vi "Read Key (Variant)__lvcfg.vi"(5 "format string (%;%f)":string="%f", 7 "section":string, 8 "error in (no error)":errorcluster, 9 "type":variant, 10 "key (optional)":string, 11 "Config in":T1) -> (0 "error out":errorcluster, 1 "key-value":variant, 2 "found?":bool, 3 "Config out":T1)   [LabVIEW 2017, in "LabVIEW Config(Variant).lvlib"]
doc: "Reads a value associated with key in a specified section of the configuration data identified by refnum. If \"key\" input is not specified, the name of the variant object is used as the key. the \"found?\" output will be TRUE for compount objects (clusters) only if all elements (recursively) are found.\n\nFor example a Boolean named \"Enable\" with a value of TRUE would correspond to the key-value pair:\n\nEnable=TRUE\n\nNote: Special characters in section and key names will be escape-coded. These include the following: \\00-\\1F (non-printable chars); \"[\", \"]\", and \"=\" (INI syntax elements); \\FE (\"þ\") and \\FF (\"ÿ\") (legacy bracket encoding); Additionally, the escape character, \"\\\", will be escaped as \"\\\\\"."
uses:
  LabVIEW Config(Variant).lvlib
  <userlib>/_NEVSTOP/Communicable State Machine(CSM)/addons/INI-Static-Variable-Support/LabVIEW-Config/Config.ctl
  <userlib>/_NEVSTOP/Communicable State Machine(CSM)/addons/INI-Static-Variable-Support/LabVIEW-Config/Read Key (String).vi
  <userlib>/_NEVSTOP/Communicable State Machine(CSM)/addons/INI-Static-Variable-Support/LabVIEW-Config/Read Key (Boolean).vi
  <userlib>/_NEVSTOP/Communicable State Machine(CSM)/addons/INI-Static-Variable-Support/LabVIEW-Config/Read Key (DBL).vi
  <userlib>/_NEVSTOP/Communicable State Machine(CSM)/addons/INI-Static-Variable-Support/LabVIEW-Config/Read Key (U32).vi
  <userlib>/_NEVSTOP/Communicable State Machine(CSM)/addons/INI-Static-Variable-Support/LabVIEW-Config/Read Key (I32).vi
  <userlib>/_NEVSTOP/Communicable State Machine(CSM)/addons/INI-Static-Variable-Support/LabVIEW-Config/LabVIEW-Config.lvlib
  <userlib>/_NEVSTOP/Communicable State Machine(CSM)/Communicable State Machine.lvlib
panel:
  in  "Ref for recursive call":refnum<vi>
  # "Read Key (Variant).vi\n\nReads a variant key-value from INI file.\n\nPlease visit http://www.OpenG.org to learn about the\nOpen Source LabVIEW software movement.\n\nNOTICE -- YOU MUST LEAVE THIS NOTICE IN PLACE.  PER THE TERMS OF THE LICENSE BELOW, YOU MAY SUBLICENSE THIS SOFTWARE \nIN ANY WAY THAT DOES NOT CONFLICT WITH THIS LICENSE.\n\n### BSD License (http://www.opensource.org/licenses/bsd-license.php) Begin ###\n \nCopyright (c) 2002, Jean-Pierre Drolet <drolet_jp@hotmail.com>\nCopyright (c) 2002-2006, Jim Kring <jim@jimkring.com>\n\nAll rights reserved.\n\nRedistribution and use in source and binary forms, with or without modification, are permitted provided that the following conditions are met:\n\n    * Redistributions of source code must retain the above copyright notice, this list of conditions and the following disclaimer.\n    * Redistributions in binary form must reproduce the above copyright notice, this list of conditions and the following disclaimer in the \n       documentation and/or other materials provided with the distribution.\n    * Neither the name of SciWare, James Kring, Inc., nor the names of its contributors may be used to endorse or promote products derived \n       from this software without specific prior written permission.\n\nTHIS SOFTWARE IS PROVIDED BY THE COPYRIGHT HOLDERS AND CONTRIBUTORS \"AS IS\" AND ANY EXPRESS OR IMPLIED WARRANTIES, \nINCLUDING, BUT NOT LIMITED TO, THE IMPLIED WARRANTIES OF MERCHANTABILITY AND FITNESS FOR A PARTICULAR PURPOSE ARE \nDISCLAIMED. IN NO EVENT SHALL THE COPYRIGHT OWNER OR CONTRIBUTORS BE LIABLE FOR ANY DIRECT, INDIRECT, INCIDENTAL,\n SPECIAL, EXEMPLARY, OR CONSEQUENTIAL DAMAGES (INCLUDING, BUT NOT LIMITED TO, PROCUREMENT OF SUBSTITUTE GOODS OR \nSERVICES; LOSS OF USE, DATA, OR PROFITS; OR BUSINESS INTERRUPTION) HOWEVER CAUSED AND ON ANY THEORY OF LIABILITY, \nWHETHER IN CONTRACT, STRICT LIABILITY, OR TORT (INCLUDING NEGLIGENCE OR OTHERWISE) ARISING IN ANY WAY OUT OF THE USE \nOF THIS SOFTWARE, EVEN IF ADVISED OF THE POSSIBILITY OF SUCH DAMAGE.\n\n### BSD License End ###"
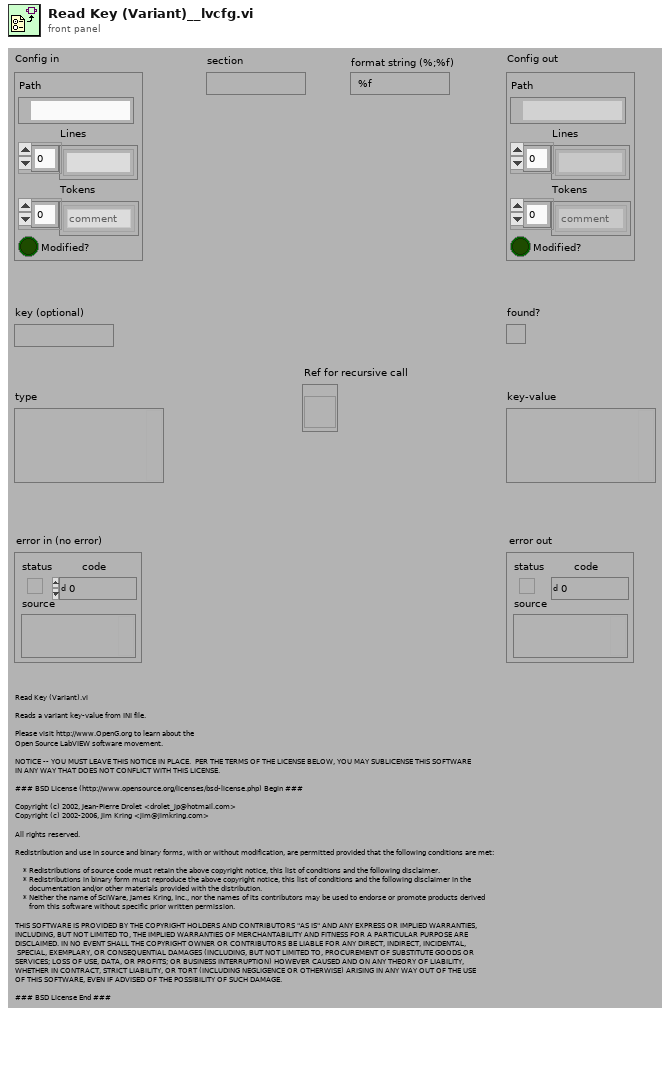
[diagram p1: front panel]
types:
  T1 = typedef "LabVIEW-Config.lvlib/Config.ctl" = cluster{"Path":path, "Lines":string[], "Tokens":enum8{"comment", "section", "key"}[], "Modified?":bool}
  T2 = typedef "Type Descriptor Enumeration__ogtk.ctl" = enum8{"<Null>", "I8", "I16", "I32", "I64", "U8", "U16", "U32", "U64", "SGL", "DBL", "EXT", "CSG", "CDB", "CXT", "0x0F", "0x10", "0x11", "0x12", "0x13", "0x14", "Enum U8", "Enum U16", "Enum U32", "Enum U64", "SGL PQ", "DBL PQ", "EXT PQ", "CSG PQ", "CDB PQ", "CXT PQ", "0x1F", "0x20", "Boolean", "0x22", "0x23", "0x24", "0x25", "0x26", "0x27", "0x28", "0x29", "0x2A", "0x2B", "0x2C", "0x2D", "0x2E", "0x2F", "String", "0x31", "Path", "Pict", "0x34", "0x35", "0x36", "DAQ", "0x38", "0x39", "0x3A", "0x3B", "0x3C", "0x3D", "0x3E", "0x3F", "Array", "0x41", "0x42", "0x43", "0x44", "0x45", "0x46", "0x47", "0x48", "0x49", "0x4A", "0x4B", "0x4C", "0x4D", "0x4E", "0x4F", "Cluster", "0x51", "0x52", "Variant", "Waveform", "0x55", "0x56", "0x57", "0x58", "0x59", "0x5A", "0x5B", "0x5C", "0x5D", "0x5E", "Fixed Point", "0x60", "0x61", "0x62", "0x63", "0x64", "0x65", "0x66", "0x67", "0x68", "0x69", "0x6A", "0x6B", "0x6C", "0x6D", "0x6E", "0x6F", "Refnum", "0x71", "0x72", "Set Collection", "Map Collection"}
  T3 = typedef "Type Descriptor__ogtk.ctl" = i16[]
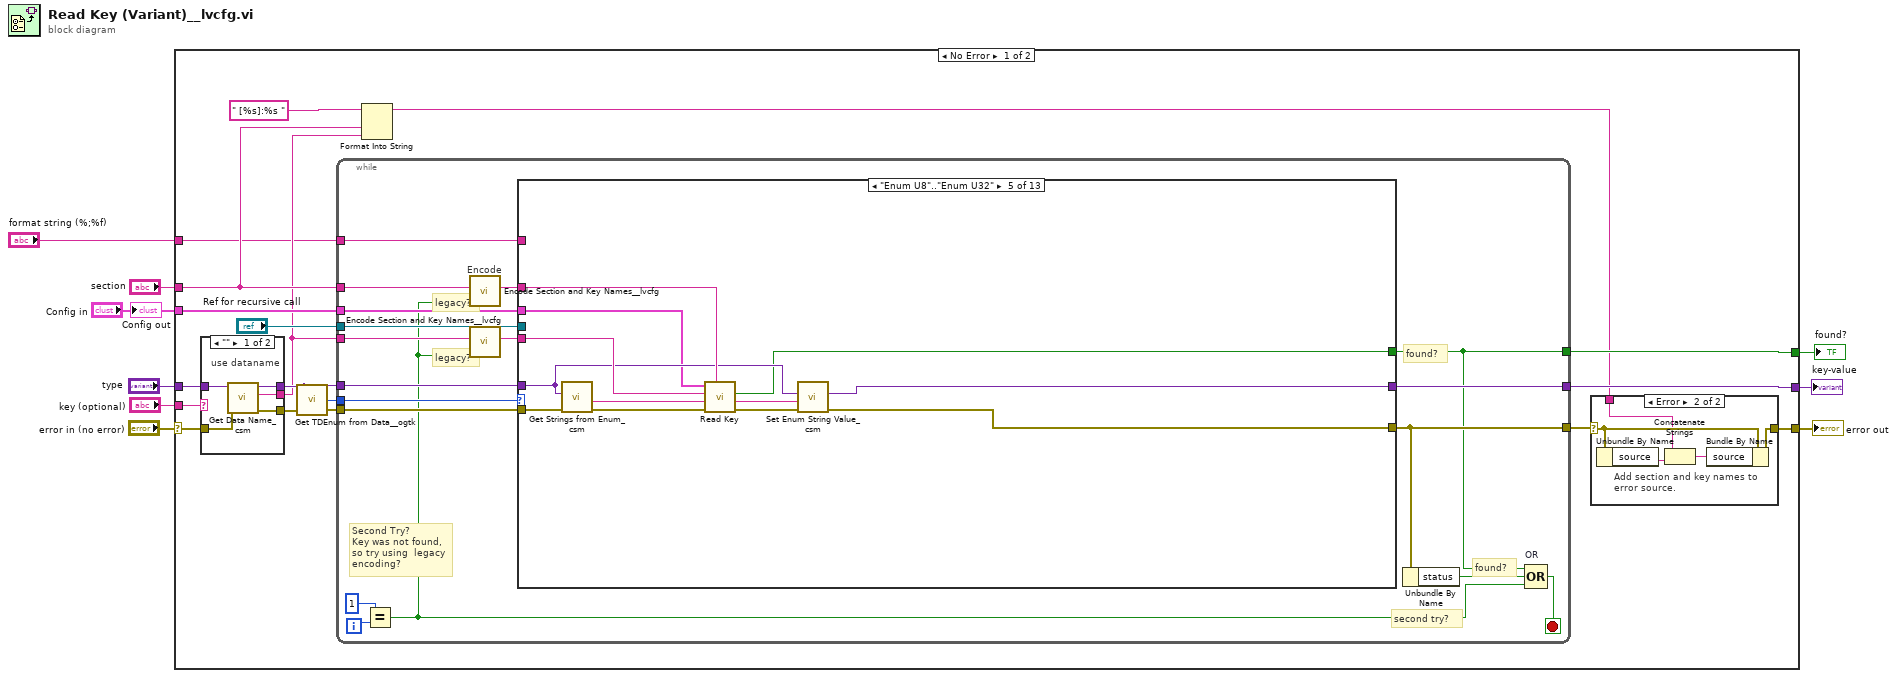
[diagram p0: block diagram]
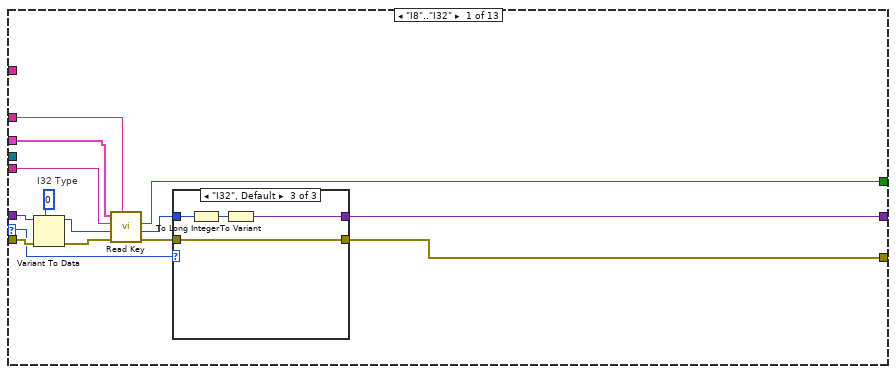
[diagram p2: hidden frame]
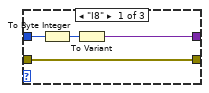
[diagram p3: hidden frame]
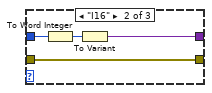
[diagram p4: hidden frame]
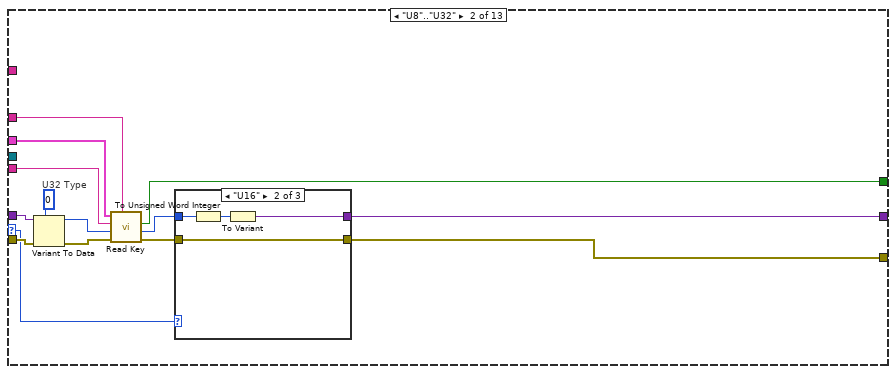
[diagram p5: hidden frame]
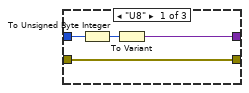
[diagram p6: hidden frame]
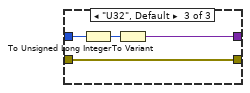
[diagram p7: hidden frame]
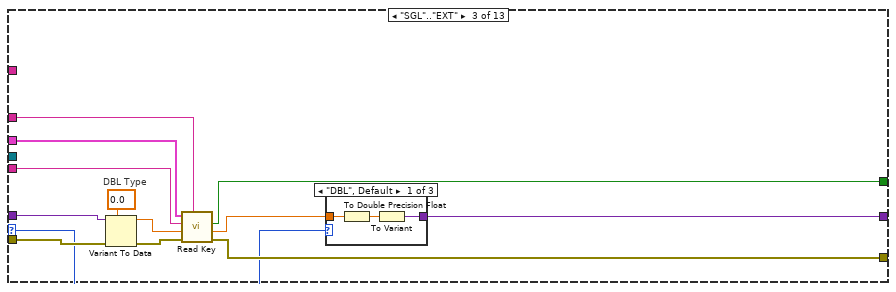
[diagram p8: hidden frame]
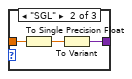
[diagram p9: hidden frame]
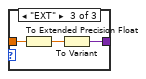
[diagram p10: hidden frame]
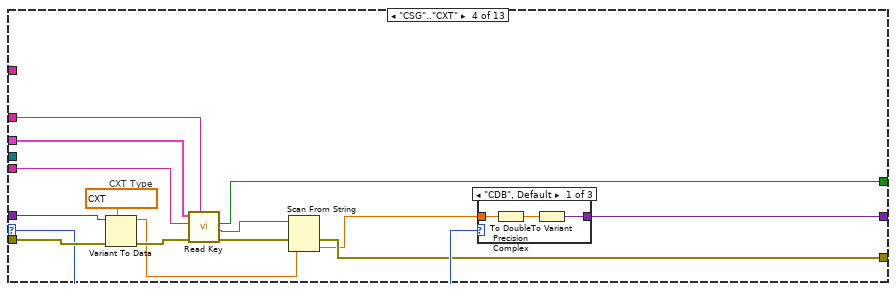
[diagram p11: hidden frame]
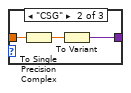
[diagram p12: hidden frame]
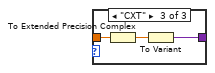
[diagram p13: hidden frame]
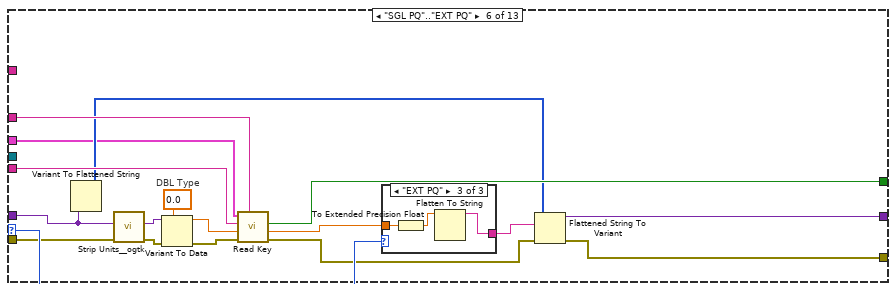
[diagram p14: hidden frame]
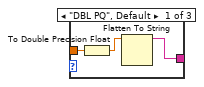
[diagram p15: hidden frame]
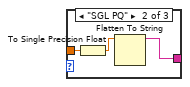
[diagram p16: hidden frame]
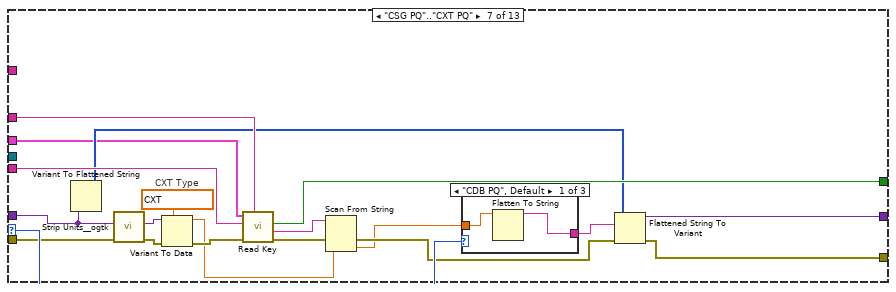
[diagram p17: hidden frame]
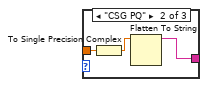
[diagram p18: hidden frame]
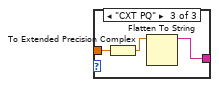
[diagram p19: hidden frame]
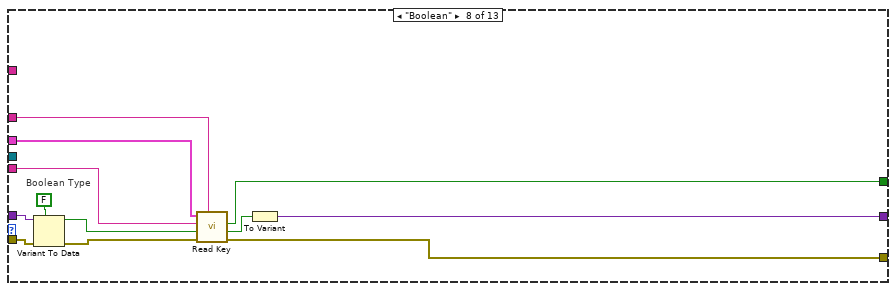
[diagram p20: hidden frame]
diagram:
  n1 = case shown="No Error" "error in (no error)" {
    selector: "error in (no error)" -> [w21 w466]
    tunnel: "Config in" -> [w25 _]
    tunnel: [w15 w466] -> w9
    tunnel: "type" -> [w23 _]
    tunnel: "key (optional)" -> [w22 _]
    tunnel: "section" -> [w12 _]
    tunnel: [w24 variant ("Variant")] -> w4
    tunnel: [w18 FALSE ("found?")] -> w2
    tunnel: "format string (%;%f)" -> [w10 _]
    frame No Error {
      n2 = case shown="\"\"" w22 {
        selector: w22 -> [_ w463]
        tunnel: [w460 w463] -> w11
        tunnel: w23 -> [w457 w461]
        tunnel: w21 -> [w459 w462]
        tunnel: [w458 w462] -> w20
        tunnel: [w456 w461] -> w19
        frame "" {
          # "use dataname"
          n3 = call <userlib>:"Get Data Name_csm.vi"("error in (no error)"=w459, "Data"=w457) -> ("error out"=w458:errorcluster, "Data Name"=w460:string, "Data dup"=w456:variant)  [unwired: 7 in]
        }
        frame Default {
          # "use optional\nkey"
        }
      }
      n4 = call <userlib>:"Get TDEnum from Data__ogtk.vi"("Data"=w19) -> ("Type Descriptor Enumeration"=w26:T2)  [unwired: 4 in]
      n5 = while {
        tunnel: w26 -> [w44]
        tunnel: w25 -> [w43]
        tunnel: [w42] -> w24
        tunnel: w20 -> [w41]
        tunnel: w19 -> [w40]
        tunnel: [w32] -> w18
        tunnel: "Ref for recursive call" -> [w39]
        tunnel: [w34] -> w16
        tunnel: w12 -> [w37]
        tunnel: w11 -> [w36]
        tunnel: w10 -> [w27]
        i -> [w31]
        stop <- w29 stop-if-true
        # "found?"
        # "found?"
        # "second try?"
        # "legacy?"
        # "legacy?"
        # "Second Try?\nKey was not found, so try using  legacy encoding?"
        # "Encode"
        n6 = Equal?(x=1, y=w31) -> (x = y?=w28:bool)
        n7 = call "Encode Section and Key Names__lvcfg.vi"("use legacy encoding scheme? (FALSE)"=w28, "string"=w37) -> ("encoded string"=w38:string)  [unwired: 9 in]
        n8 = call "Encode Section and Key Names__lvcfg.vi"("use legacy encoding scheme? (FALSE)"=w28, "string"=w36) -> ("encoded string"=w35:string)  [unwired: 9 in]
        n9 = case shown="\"Enum U8\"..\"Enum U32\"" w44 {
          selector: w44 -> [w49 w75 w98 w125 _ w165 w196 _ _ _ _ _ _]
          tunnel: w40 -> [w57 w83 w108 w132 w146 w158 w190 w220 w232 w244 w248 w396 w447]
          tunnel: w43 -> [w45 w72 w97 w119 w143 w155 w182 w210 w222 w235 w255 w410 w437]
          tunnel: [w48 w73 w106 w123 w148 w160 w192 w218 w230 w242 w252 w399 w442] -> w34
          tunnel: w41 -> [w55 w81 w105 w130 w152 w164 w195 w217 w229 w241 w258 w398 w444]
          tunnel: w35 -> [w54 w80 w104 w129 w154 w170 w199 w216 w228 w240 w249 w408 w449]
          tunnel: w38 -> [w53 w79 w103 w128 w153 w169 w198 w215 w227 w239 w250 w409 w448]
          tunnel: [w47 w77 w100 w127 w145 w156 w188 w212 w226 w237 w253 w400 w445] -> w42
          tunnel: [w52 w76 w99 w126 w144 w166 w197 w211 w224 w236 w251 w404 w440] -> w32
          tunnel: w39 -> [_ _ _ _ _ _ _ _ _ _ w254 w403 _]
          tunnel: w27 -> [_ _ _ _ _ _ _ _ _ _ w246 w393 _]
          frame "I8".."I32" {
            # "I32 Type"
            n10 = Variant To Data(error in=w55, type=0, Variant=w57) -> (data=w46:i32, error out=w56:errorcluster)
            n11 = call-poly <userlib>:"Read Key.vi"("Section Name"=w53, "error in (no error)"=w56, "Default"=w46, "Key Name"=w54, "Config in"=w45) -> ("error out"=w51:errorcluster, "Value"=w50:i32, "Key Found?"=w52:bool)  [unwired: 3 in, 1 out]
            n12 = case shown="\"I32\", Default" w49 {
              tunnel: w50 -> [w62 w66 w70]
              tunnel: [w61 w65 w69] -> w47
              tunnel: w51 -> [w59 w63 w67]
              tunnel: [w59 w63 w67] -> w48
              frame "I8" {
                n13 = To Byte Integer(number=w62) -> (8bit integer=w60:i8)
                n14 = To Variant(anything=w60) -> (Variant=w61:variant)
              }
              frame "I16" {
                n15 = To Word Integer(number=w66) -> (16bit integer=w64:i16)
                n16 = To Variant(anything=w64) -> (Variant=w65:variant)
              }
              frame "I32", Default {
                n17 = To Long Integer(number=w70) -> (32bit integer=w68:i32)
                n18 = To Variant(anything=w68) -> (Variant=w69:variant)
              }
            }
          }
          frame "U8".."U32" {
            # "U32 Type"
            n19 = Variant To Data(error in=w81, type=u32 0, Variant=w83) -> (data=w71:u32, error out=w82:errorcluster)
            n20 = call-poly <userlib>:"Read Key.vi"("Section Name"=w79, "error in (no error)"=w82, "Default"=w71, "Key Name"=w80, "Config in"=w72) -> ("error out"=w74:errorcluster, "Value"=w78:u32, "Key Found?"=w76:bool)  [unwired: 3 in, 1 out]
            n21 = case shown="\"U16\"" w75 {
              tunnel: w78 -> [w88 w92 w96]
              tunnel: [w87 w91 w95] -> w77
              tunnel: w74 -> [w85 w89 w93]
              tunnel: [w85 w89 w93] -> w73
              frame "U8" {
                n22 = To Unsigned Byte Integer(number=w88) -> (unsigned 8bit integer=w86:u8)
                n23 = To Variant(anything=w86) -> (Variant=w87:variant)
              }
              frame "U16" {
                n24 = To Unsigned Word Integer(number=w92) -> (unsigned 16bit integer=w90:u16)
                n25 = To Variant(anything=w90) -> (Variant=w91:variant)
              }
              frame "U32", Default {
                n26 = To Unsigned Long Integer(number=w96) -> (unsigned 32bit integer=w94:u32)
                n27 = To Variant(anything=w94) -> (Variant=w95:variant)
              }
            }
          }
          frame "SGL".."EXT" {
            # "DBL Type"
            n28 = Variant To Data(error in=w105, type=0.0, Variant=w108) -> (data=w102:dbl, error out=w107:errorcluster)
            n29 = call-poly <userlib>:"Read Key.vi"("Section Name"=w103, "error in (no error)"=w107, "Default"=w102, "Key Name"=w104, "Config in"=w97) -> ("error out"=w106:errorcluster, "Value"=w101:dbl, "Key Found?"=w99:bool)  [unwired: 3 in, 1 out]
            n30 = case shown="\"DBL\", Default" w98 {
              tunnel: w101 -> [w112 w115 w118]
              tunnel: [w111 w114 w117] -> w100
              frame "DBL", Default {
                n31 = To Double Precision Float(number=w112) -> (double precision float=w110:dbl)
                n32 = To Variant(anything=w110) -> (Variant=w111:variant)
              }
              frame "SGL" {
                n33 = To Single Precision Float(number=w115) -> (single precision float=w113:sgl)
                n34 = To Variant(anything=w113) -> (Variant=w114:variant)
              }
              frame "EXT" {
                n35 = To Extended Precision Float(1:w118) -> (0:w116:ext)
                n36 = To Variant(anything=w116) -> (Variant=w117:variant)
              }
            }
          }
          frame "CSG".."CXT" {
            # "CXT Type"
            n37 = Variant To Data(error in=w130, type=cxt 0.0+0.0i, Variant=w132) -> (data=w121:cxt, error out=w131:errorcluster)
            n38 = call-poly <userlib>:"Read Key.vi"("Section Name"=w128, "error in (no error)"=w131, "Key Name"=w129, "Config in"=w119) -> ("error out"=w124:errorcluster, "Value"=w122:string, "Key Found?"=w126:bool)  [unwired: 4 in, 1 out]
            n39 = Scan From String(input string=w122, error in=w124, default 1=w121) -> (error out=w123:errorcluster, output 1=w120:cxt)  [unwired: 2 in, 2 out]
            n40 = case shown="\"CDB\", Default" w125 {
              tunnel: w120 -> [w136 w139 w142]
              tunnel: [w135 w138 w141] -> w127
              frame "CDB", Default {
                n41 = To Double Precision Complex(1:w136) -> (0:w134:cdb)
                n42 = To Variant(anything=w134) -> (Variant=w135:variant)
              }
              frame "CSG" {
                n43 = To Single Precision Complex(1:w139) -> (0:w137:csg)
                n44 = To Variant(anything=w137) -> (Variant=w138:variant)
              }
              frame "CXT" {
                n45 = To Extended Precision Complex(1:w142) -> (0:w140:cxt)
                n46 = To Variant(anything=w140) -> (Variant=w141:variant)
              }
            }
          }
          frame "Enum U8".."Enum U32" {
            n47 = call <userlib>:"Get Strings from Enum_csm.vi"("error in (no error)"=w152, "Enum"=w146) -> ("error out"=w151:errorcluster, "String Value"=w150:string)  [unwired: 6 in, 2 out]
            n48 = call-poly <userlib>:"Read Key.vi"("Section Name"=w153, "error in (no error)"=w151, "Default"=w150, "Key Name"=w154, "Config in"=w143) -> ("error out"=w149:errorcluster, "Value"=w147:string, "Key Found?"=w144:bool)  [unwired: 3 in, 1 out]
            n49 = call <userlib>:"Set Enum String Value_csm.vi"("error in (no error)"=w149, "String Value"=w147, "Default Enum Value"=w146) -> ("error out"=w148:errorcluster, "Enum"=w145:variant)  [unwired: 7 in]
          }
          frame "SGL PQ".."EXT PQ" {
            # "DBL Type"
            n50 = Variant To Flattened String(Variant=w158) -> (1:w157:i16[])  [unwired: 1 out]
            n51 = call <userlib>:"Strip Units__ogtk.vi"("error in (no error)"=w164, "Number or 1D array with units"=w158) -> ("error out"=w162:errorcluster, "Pure Number(s) (base units)"=w163:variant)  [unwired: 8 in]
            n52 = Variant To Data(error in=w162, type=0.0, Variant=w163) -> (data=w168:dbl, error out=w171:errorcluster)
            n53 = call-poly <userlib>:"Read Key.vi"("Section Name"=w169, "error in (no error)"=w171, "Default"=w168, "Key Name"=w170, "Config in"=w155) -> ("error out"=w161:errorcluster, "Value"=w167:dbl, "Key Found?"=w166:bool)  [unwired: 3 in, 1 out]
            n54 = case shown="\"EXT PQ\"" w165 {
              tunnel: w167 -> [w175 w178 w181]
              tunnel: [w174 w176 w179] -> w159
              frame "DBL PQ", Default {
                n55 = To Double Precision Float(number=w175) -> (double precision float=w173:dbl)
                n56 = Flatten To String(anything=w173) -> (data string=w174:string)  [unwired: 3 in, 2 out]
              }
              frame "SGL PQ" {
                n57 = To Single Precision Float(number=w178) -> (single precision float=w177:sgl)
                n58 = Flatten To String(anything=w177) -> (data string=w176:string)  [unwired: 3 in, 2 out]
              }
              frame "EXT PQ" {
                n59 = To Extended Precision Float(1:w181) -> (0:w180:ext)
                n60 = Flatten To String(anything=w180) -> (data string=w179:string)  [unwired: 3 in, 2 out]
              }
            }
            n61 = Flattened String To Variant(4:w161, 6:w159, 7:w157) -> (0:w160:errorcluster, 3:w156:variant)
          }
          frame "CSG PQ".."CXT PQ" {
            # "CXT Type"
            n62 = Variant To Flattened String(Variant=w190) -> (1:w189:i16[])  [unwired: 1 out]
            n63 = call <userlib>:"Strip Units__ogtk.vi"("error in (no error)"=w195, "Number or 1D array with units"=w190) -> ("error out"=w193:errorcluster, "Pure Number(s) (base units)"=w194:variant)  [unwired: 8 in]
            n64 = Variant To Data(error in=w193, type=cxt 0.0+0.0i, Variant=w194) -> (data=w184:cxt, error out=w200:errorcluster)
            n65 = call-poly <userlib>:"Read Key.vi"("Section Name"=w198, "error in (no error)"=w200, "Key Name"=w199, "Config in"=w182) -> ("error out"=w186:errorcluster, "Value"=w185:string, "Key Found?"=w197:bool)  [unwired: 4 in, 1 out]
            n66 = Scan From String(input string=w185, error in=w186, default 1=w184) -> (error out=w187:errorcluster, output 1=w183:cxt)  [unwired: 2 in, 2 out]
            n67 = case shown="\"CDB PQ\", Default" w196 {
              tunnel: w183 -> [w203 w206 w209]
              tunnel: [w202 w204 w207] -> w191
              frame "CDB PQ", Default {
                n68 = Flatten To String(anything=w203) -> (data string=w202:string)  [unwired: 3 in, 2 out]
              }
              frame "CSG PQ" {
                n69 = To Single Precision Complex(1:w206) -> (0:w205:csg)
                n70 = Flatten To String(anything=w205) -> (data string=w204:string)  [unwired: 3 in, 2 out]
              }
              frame "CXT PQ" {
                n71 = To Extended Precision Complex(1:w209) -> (0:w208:cxt)
                n72 = Flatten To String(anything=w208) -> (data string=w207:string)  [unwired: 3 in, 2 out]
              }
            }
            n73 = Flattened String To Variant(4:w187, 6:w191, 7:w189) -> (0:w192:errorcluster, 3:w188:variant)
          }
          frame "Boolean" {
            # "Boolean Type"
            n74 = Variant To Data(error in=w217, type=FALSE, Variant=w220) -> (data=w214:bool, error out=w219:errorcluster)
            n75 = call-poly <userlib>:"Read Key.vi"("Section Name"=w215, "error in (no error)"=w219, "Default"=w214, "Key Name"=w216, "Config in"=w210) -> ("error out"=w218:errorcluster, "Value"=w213:bool, "Key Found?"=w211:bool)  [unwired: 3 in, 1 out]
            n76 = To Variant(anything=w213) -> (Variant=w212:variant)
          }
          frame "String", "DAQ" {
            # "String Type"
            n77 = Variant To Data(error in=w229, type="", Variant=w232) -> (data=w223:string, error out=w231:errorcluster)
            n78 = call-poly <userlib>:"Read Key.vi"("Section Name"=w227, "error in (no error)"=w231, "Default"=w223, "Key Name"=w228, "Config in"=w222) -> ("error out"=w230:errorcluster, "Value"=w225:string, "Key Found?"=w224:bool)  [unwired: 3 in, 1 out]
            n79 = To Variant(anything=w225) -> (Variant=w226:variant)
          }
          frame "Path" {
            # "Path Type"
            n80 = Variant To Data(error in=w241, type=path "", Variant=w244) -> (error out=w243:errorcluster)  [unwired: 1 out]
            n81 = call-poly <userlib>:"Read Key.vi"("Section Name"=w239, "error in (no error)"=w243, "Key Name"=w240, "Config in"=w235) -> ("error out"=w242:errorcluster, "Value"=w238:string, "Key Found?"=w236:bool)  [unwired: 4 in, 1 out]
            n82 = String To Path(string=w238) -> (path=w234:path)
            n83 = To Variant(anything=w234) -> (Variant=w237:variant)
          }
          frame "Array" {
            n84 = call <userlib>:"Reshape Array to 1D VArray__ogtk.vi"("error in (no error)"=w258, "MultiD Array"=w248) -> ("error out"=w259:errorcluster, "1D VArray"=w247:variant)  [unwired: 7 in, 1 out]
            n85 = call <userlib>:"Get Array Element TDEnum__ogtk.vi"("error in (no error)"=w259, "Array"=w247) -> ("error out"=w256:errorcluster, "Element Type"=w257:T2)  [unwired: 8 in]
            n86 = case shown="Default" w257 {
              selector: w257 -> [_ w341]
              tunnel: w256 -> [_ w351]
              tunnel: w248 -> [w270 w329]
              tunnel: w250 -> [w268 w352]
              tunnel: w255 -> [w261 w324]
              tunnel: w249 -> [w271 w325]
              tunnel: w254 -> [w269 _]
              tunnel: [w266 w328] -> w253
              tunnel: [w265 errorcluster {"status"=FALSE, "code"=0, "source"=""} ("error out")] -> w252
              tunnel: [w264 w350] -> w251
              tunnel: w246 -> [w262 w326]
              frame Default {
                n87 = Concatenate Strings(w271, ".<size(s)>" ("Substring")) -> (w274:string)
                n88 = call-poly <userlib>:"Read Key.vi"("Read Raw String? (F)"=TRUE ("read raw string? (F)"), "Section Name"=w268, "Key Name"=w274, "Config in"=w261) -> ("error out"=w272:errorcluster, "Value"=w273:string, "Key Found?"=w263:bool, "Config out"=w260:T1)  [unwired: 4 in]
                n89 = case shown="True" w263 {
                  tunnel: w273 -> [_ w305]
                  tunnel: w272 -> [_ w281]
                  tunnel: w271 -> [_ w300]
                  tunnel: w270 -> [w277 w299]
                  tunnel: w269 -> [_ w298]
                  tunnel: w268 -> [_ w296]
                  tunnel: w260 -> [_ w295]
                  tunnel: [w277 w288] -> w266
                  tunnel: [errorcluster {"status"=FALSE, "code"=0, "source"=""} ("error out") w287] -> w265
                  tunnel: [FALSE w285] -> w264
                  tunnel: w262 -> [_ w279]
                  frame False {
                    # "array size(s) not found. Ignore element keys (if any) and return input array"
                  }
                  frame True {
                    # "array.size(s) is found. Read elements keys. missing keys replace with datatype default."
                    n90 = call <userlib>:"Get Array Element TD__ogtk.vi"("error in (no error)"=w281, "Array"=w299) -> ("error out"=w283:errorcluster, "Type Descriptor"=w284:T3)  [unwired: 8 in]
                    n91 = property class="VI"() -> ("VI Name"=w302:string)  [unwired: 2 in, 2 out]
                    n92 = call <userlib>:"Get Default Data from TD__ogtk.vi"("error in (no error)"=w283, "Type Descriptor"=w284) -> ("error out"=w280:errorcluster, "Default VData"=w282:variant)  [unwired: 8 in]
                    n93 = Spreadsheet String To Array(delimiter (Tab)=" ", format string="%d", spreadsheet string=w305, array type (2D Dbl)=u32[] [] ("Array Constant")) -> (array=w289:u32[])
                    n94 = Open VI Reference(type specifier VI Refnum (for type only)=w298, vi path=w302, error in (no error)=w280) -> (vi reference=w297:refnum<vi>, error out=w301:errorcluster)  [unwired: 3 in]
                    n95 = Multiply Array Elements(1:w289) -> (0:w303:u32)
                    n96 = for {
                      N: w303 -> [_]
                      shift-right: [w317] -> w292
                      shift-left: w301 -> [w314]
                      shift-right: [w318] -> w294
                      shift-left: w297 -> [w316]
                      tunnel: w300 -> [w321]
                      tunnel: w282 -> [w315]
                      tunnel: w296 -> [w312]
                      tunnel: w295 -> [w308]
                      tunnel: [w311] -> w293 mode=indexing
                      tunnel: [w310] -> w286 mode=indexing
                      tunnel: w279 -> [w309]
                      i -> [w322]
                      n97 = Format Into String(format string=" %d" ("Format String"), initial string=w321, w322) -> (resulting string=w313:string)  [unwired: 1 in, 1 out]
                      n98 = call-by-ref "?"(reference=w316, error in=w314, "format string (%;%f)"=w309, "section"=w312, "type"=w315, "key (optional)"=w313, "Config in"=w308) -> (reference out=w318:refnum<vi>, error out=w320:errorcluster, "error out"=w319:errorcluster, "key-value"=w311:variant, "found?"=w310:bool)  [unwired: 3 in, 1 out]
                      n99 = Merge Errors(w320, w319) -> (w317:errorcluster)
                    }
                    n100 = And Array Elements(Boolean array=w286) -> (logical AND=w285:bool)
                    n101 = Close Reference(reference=w294) -> ()  [unwired: 1 in, 1 out]
                    n102 = call <userlib>:"Array of VData to VArray__ogtk.vi"("error in (no error)"=w292, "Element Type (when empty)"=w282, "1D Array of VData"=w293) -> ("error out"=w291:errorcluster, "VArray"=w290:variant)  [unwired: 7 in]
                    n103 = call <userlib>:"Reshape 1D Array__ogtk.vi"("error in (no error)"=w291, "Size(s)"=w289, "1D Array"=w290) -> ("error out"=w287:errorcluster, "Reshaped VArray"=w288:variant)  [unwired: 7 in]
                  }
                }
              }
              frame "I8".."I32", "U8".."U32", "SGL".."EXT", "SGL PQ".."EXT PQ" {
                n104 = call-poly <userlib>:"Read Key.vi"("Section Name"=w352, "error in (no error)"=w351, "Key Name"=w325, "Config in"=w324) -> ("error out"=w349:errorcluster, "Value"=w353:string, "Key Found?"=w350:bool)  [unwired: 4 in, 1 out]
                n105 = Scan From String(format string="<size(s)=%[\\s0-9]> " ("regular expression"), input string=w353, error in=w349) -> (remaining string=w342:string, error out=w332:errorcluster, output 1=w347:string)  [unwired: 2 in, 1 out]
                n106 = Variant To Flattened String(Variant=w329) -> (data string=w334:string, 1:w335:i16[])
                n107 = Spreadsheet String To Array(delimiter (Tab)=" ", format string="%d", spreadsheet string=w347, array type (2D Dbl)=u32[] []) -> (array=w348:u32[])
                n108 = Type Cast(x=w348) -> (*(type *) &x=w339:string)  [unwired: 1 in]
                n109 = Spreadsheet String To Array(delimiter (Tab)=" ", format string=w326, spreadsheet string=w342, array type (2D Dbl)=dbl[] []) -> (array=w340:dbl[])
                n110 = case shown="\"SGL\", \"SGL PQ\"" w341 {
                  tunnel: w340 -> [_ w360 w364 w368 w372 w376 w380 w384 w386 w390]
                  tunnel: [w355 w358 w362 w366 w370 w374 w378 w382 w388 w392] -> w337
                  tunnel: ["" w357 w361 w365 w369 w373 w377 w381 w387 w391] -> w336
                  tunnel: w339 -> [_ w357 w361 w365 w369 w373 w377 w381 w387 w391]
                  tunnel: w334 -> [w355 _ _ _ _ _ _ _ _ _]
                  frame Default {
                  }
                  frame "I8" {
                    n111 = To Byte Integer(number=w360) -> (8bit integer=w359:i8[])
                    n112 = Type Cast(x=w359) -> (*(type *) &x=w358:string)  [unwired: 1 in]
                  }
                  frame "I16" {
                    n113 = To Word Integer(number=w364) -> (16bit integer=w363:i16[])
                    n114 = Type Cast(x=w363) -> (*(type *) &x=w362:string)  [unwired: 1 in]
                  }
                  frame "I32" {
                    n115 = To Long Integer(number=w368) -> (32bit integer=w367:i32[])
                    n116 = Type Cast(x=w367) -> (*(type *) &x=w366:string)  [unwired: 1 in]
                  }
                  frame "U8" {
                    n117 = To Unsigned Byte Integer(number=w372) -> (unsigned 8bit integer=w371:u8[])
                    n118 = Type Cast(x=w371) -> (*(type *) &x=w370:string)  [unwired: 1 in]
                  }
                  frame "U16" {
                    n119 = To Unsigned Word Integer(number=w376) -> (unsigned 16bit integer=w375:u16[])
                    n120 = Type Cast(x=w375) -> (*(type *) &x=w374:string)  [unwired: 1 in]
                  }
                  frame "U32" {
                    n121 = To Unsigned Long Integer(number=w380) -> (unsigned 32bit integer=w379:u32[])
                    n122 = Type Cast(x=w379) -> (*(type *) &x=w378:string)  [unwired: 1 in]
                  }
                  frame "SGL", "SGL PQ" {
                    n123 = To Single Precision Float(number=w384) -> (single precision float=w383:sgl[])
                    n124 = Type Cast(x=w383) -> (*(type *) &x=w382:string)  [unwired: 1 in]
                  }
                  frame "DBL", "DBL PQ" {
                    n125 = To Double Precision Float(number=w386) -> (double precision float=w385:dbl[])
                    n126 = Type Cast(x=w385) -> (*(type *) &x=w388:string)  [unwired: 1 in]
                  }
                  frame "EXT", "EXT PQ" {
                    n127 = To Extended Precision Float(1:w390) -> (0:w389:ext[])
                    n128 = Type Cast(x=w389) -> (*(type *) &x=w392:string)  [unwired: 1 in]
                  }
                }
                n129 = Concatenate Strings(w336, w337) -> (w338:string)
                n130 = Flattened String To Variant(4:w332, 6:w338, 7:w335) -> (0:w331:errorcluster, 3:w330:variant)
                n131 = Select(t=w329, s=w331, f=w330) -> (s? t:f=w328:variant)
              }
            }
          }
          frame "Cluster" {
            # ">> Cluster Name >>"
            # "Expand cluster to its elements\nand read keys recursively."
            n132 = call <userlib>:"Get Data Name_csm.vi"("error in (no error)"=w398, "Data"=w396) -> ("error out"=w397:errorcluster, "Data Name"=w394:string, "Data dup"=w395:variant)  [unwired: 7 in]
            n133 = call <userlib>:"Cluster to Array of VData__ogtk.vi"("error in (no error)"=w397, "Cluster"=w395) -> ("error out"=w416:errorcluster, "Array of VData"=w415:variant[])  [unwired: 8 in]
            n134 = property class="VI"() -> ("VI Name"=w414:string)  [unwired: 2 in, 2 out]
            n135 = Open VI Reference(type specifier VI Refnum (for type only)=w403, vi path=w414, error in (no error)=w416) -> (vi reference=w411:refnum<vi>, error out=w413:errorcluster)  [unwired: 3 in]
            n136 = for {
              shift-right: [w435] -> w412
              shift-left: w411 -> [w436]
              shift-right: [w421] -> w406
              shift-left: w413 -> [w431]
              tunnel: w415 -> [w429] mode=indexing
              tunnel: w409 -> [w426]
              tunnel: w410 -> [w417]
              tunnel: w408 -> [w433]
              tunnel: [w423] -> w407 mode=indexing
              tunnel: [w419] -> w405 mode=indexing
              tunnel: w393 -> [w418]
              n137 = call <userlib>:"Get Data Name_csm.vi"("error in (no error)"=w431, "Data"=w429) -> ("error out"=w430:errorcluster, "Data Name"=w420:string, "Data dup"=w428:variant)  [unwired: 7 in]
              n138 = Format Into String(format string=".%s" ("Format String"), initial string=w433, w420) -> (resulting string=w427:string)  [unwired: 1 in, 1 out]
              n139 = call-by-ref "?"(reference=w436, error in=w430, "format string (%;%f)"=w418, "section"=w426, "type"=w428, "key (optional)"=w427, "Config in"=w417) -> (reference out=w435:refnum<vi>, error out=w434:errorcluster, "error out"=w425:errorcluster, "key-value"=w424:variant, "found?"=w419:bool)  [unwired: 3 in, 1 out]
              n140 = Merge Errors(w434, w425) -> (w422:errorcluster)
              n141 = call <userlib>:"Set Data Name_csm.vi"("error in (no error)"=w422, "Data Name"=w420, "Data"=w424) -> ("error out"=w421:errorcluster, "Renamed Data"=w423:variant)  [unwired: 7 in]
            }
            n142 = And Array Elements(Boolean array=w405) -> (logical AND=w404:bool)
            n143 = call <userlib>:"Array of VData to VCluster__ogtk.vi"("error in (no error)"=w406, "Array"=w407) -> ("error out"=w402:errorcluster, "VCluster"=w401:variant)  [unwired: 8 in]
            n144 = Close Reference(reference=w412) -> ()  [unwired: 1 in, 1 out]
            n145 = call <userlib>:"Set Data Name_csm.vi"("error in (no error)"=w402, "Data Name"=w394, "Data"=w401) -> ("error out"=w399:errorcluster, "Renamed Data"=w400:variant)  [unwired: 7 in]
          }
          frame Default {
            n146 = Variant To Flattened String(Variant=w447) -> (data string=w439:string, 1:w441:i16[])
            n147 = call-poly <userlib>:"Read Key.vi"("Read Raw String? (F)"=TRUE, "Section Name"=w448, "error in (no error)"=w444, "Default"=w439, "Key Name"=w449, "Config in"=w437) -> ("error out"=w443:errorcluster, "Value"=w446:string, "Key Found?"=w440:bool)  [unwired: 2 in, 1 out]
            n148 = Flattened String To Variant(4:w443, 6:w446, 7:w441) -> (0:w442:errorcluster, 3:w445:variant)
          }
        }
        n149 = Unbundle By Name(w34) -> ("status"=w33:bool)
        n150 = Compound Arithmetic op=OR "OR"(w32, w33, w28) -> (w29:bool)
      }
      n151 = Format Into String(format string=" [%s]:%s " ("Format String"), w12, w11) -> (resulting string=w13:string)  [unwired: 2 in, 1 out]
      n152 = case shown="Error" w16 {
        selector: w16 -> [w450 w455]
        tunnel: [w450 w454] -> w15
        tunnel: w13 -> [_ w451]
        frame No Error {
        }
        frame Error {
          # "Add section and key names to\nerror source."
          n153 = Unbundle By Name(w455) -> ("source"=w452:string)
          n154 = Concatenate Strings(w451, w452) -> (w453:string)
          n155 = Bundle By Name(cluster=w455, "source"=w453) -> (w454:errorcluster)
        }
      }
    }
    frame Error {
    }
  }
  "error out" <- w9
  "key-value" <- w4
  "found?" <- w2
  "Config out" <- "Config in"
